vi "get queues.vi"(11 "error in (no error)":errorcluster) -> (4 "display queues":T1, 8 "disk queues":T1, 15 "error out":errorcluster)   [LabVIEW 2017]
uses:
  typedefs/queue cluster.ctl
  typedefs/reading queue.ctl
  typedefs/reading.ctl
  typedefs/readingType.ctl
  typedefs/magnetomter reading set.ctl
  popup panels/control panel globals.vi
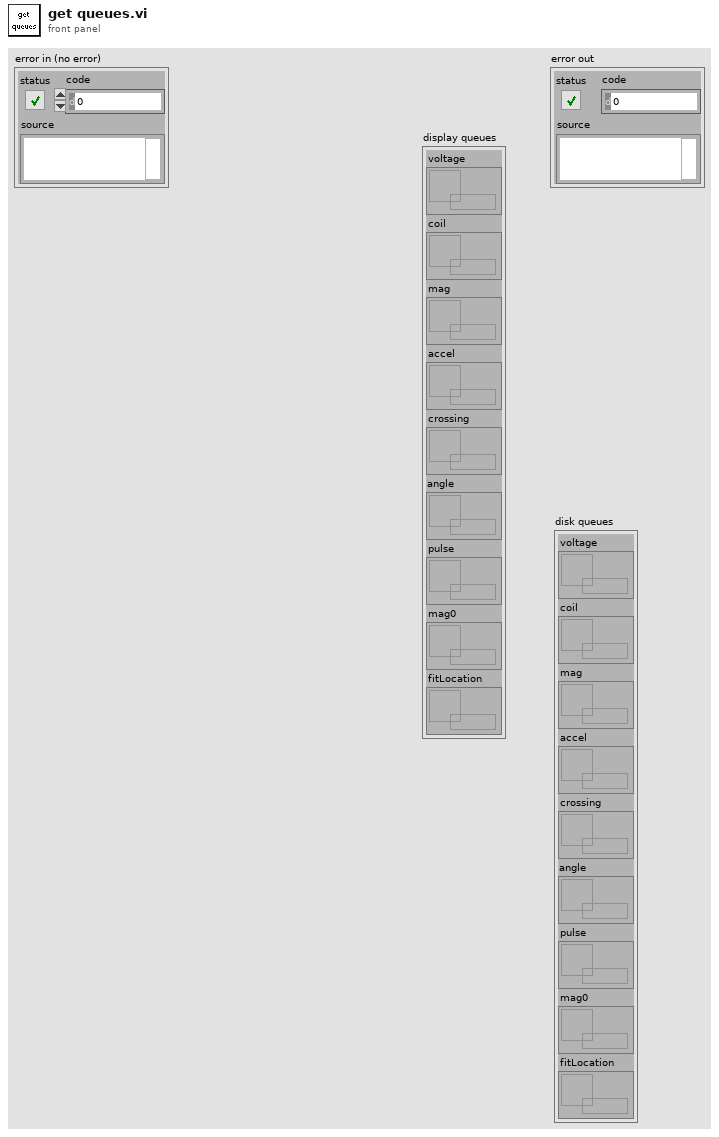
[diagram p1: front panel]
types:
  T1 = typedef "queue cluster.ctl" = cluster{"voltage":T2, "coil":T2, "mag":refnum<queue>, "accel":T2, "crossing":T2, "angle":T2, "pulse":T2, "mag0":T2, "fitLocation":T2}
  T2 = typedef "reading queue.ctl" = refnum<queue>
  T3 = typedef "magnetomter reading set.ctl" = cluster{"time":fxp<+,48,48>, "mag readings":cluster{"magnetometer index":dbl, "Bx":dbl, "By":dbl, "Bz":dbl, "magnetometer x":dbl, "magnetometer y":dbl}[]}
  T4 = typedef "reading.ctl" = cluster{"reading type":T5, "time":fxp<+,48,48>, "x":sgl, "y":sgl, "z":sgl, "XSUM":u8}
  T5 = typedef "readingType.ctl" = enum8{"SYNC", "DETVAL", "COILI", "MAGVEC", "ACCVEC", "CROSSING", "MAGVEC0", "MAGVEC1", "MAGVEC2", "MAGVEC3", "MAGVEC4", "MAGVEC5", "MAGVEC6", "MAGVEC7"}
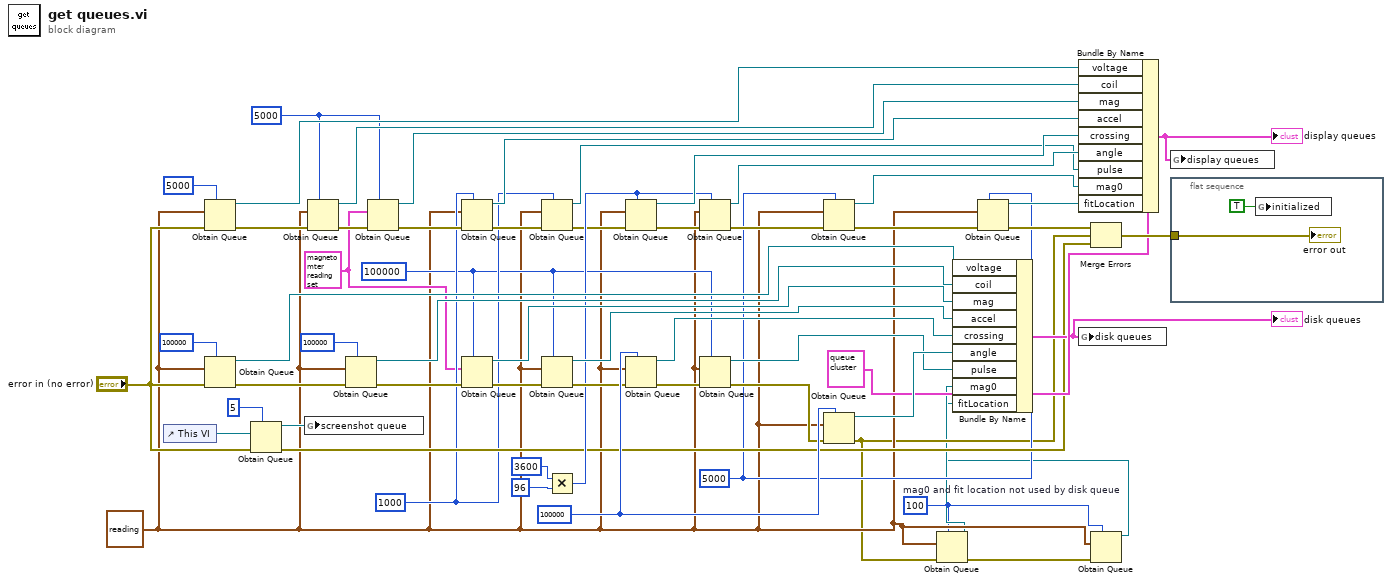
[diagram p0: block diagram]
diagram:
  w1 = 100  # mag0 and fit location not used by disk queue
  w7 = 5000 ("max queue size (-1, unlimited)")
  w13 = T3 {"time"=0.0, "mag readings"=[]} ("Magnetometer reading set")
  w32 = T1 {"voltage"=refnum, "coil"=refnum, "mag"=refnum, "accel"=refnum, "crossing"=refnum, "angle"=refnum, "pulse"=refnum, "mag0"=refnum, "fitLocation"=refnum} ("queue cluster")
  w36 = 100000 ("max queue size (-1, unlimited)")
  w15 = 100000 ("max queue size (-1, unlimited)")
  w19 = 1000 ("max queue size (-1, unlimited)")
  w6 = T4 {"reading type"=enum."SYNC", "time"=0.0, "x"=0.0, "y"=0.0, "z"=0.0, "XSUM"=0} ("reading3")
  w31 = 5000 ("max queue size (-1, unlimited)")
  n1 = control-ref of="This VI"() -> (w24:refnum<vi>)
  n2 = Obtain Queue(max queue size (-1, unlimited)=5000, element data type=w6, error in (no error)="error in (no error)") -> (queue out=w54:refnum<queue>, error out=w57:errorcluster)  [unwired: 2 in, 1 out]
  n3 = Obtain Queue(max queue size (-1, unlimited)=100000, element data type=w6, error in (no error)="error in (no error)") -> (queue out=w45:refnum<queue>, error out=w48:errorcluster)  [unwired: 2 in, 1 out]
  n4 = Obtain Queue(max queue size (-1, unlimited)=5, element data type=w24, error in (no error)="error in (no error)") -> (queue out=w22:refnum<queue>, error out=w23:errorcluster)  [unwired: 2 in, 1 out]
  n5 = global write "control panel globals.vi" "screenshot queue"(w22) -> ()
  n6 = Obtain Queue(max queue size (-1, unlimited)=w31, element data type=w6, error in (no error)=w57) -> (queue out=w53:refnum<queue>, error out=w56:errorcluster)  [unwired: 2 in, 1 out]
  n7 = Obtain Queue(max queue size (-1, unlimited)=100000, element data type=w6, error in (no error)=w48) -> (queue out=w44:refnum<queue>, error out=w47:errorcluster)  [unwired: 2 in, 1 out]
  n8 = Obtain Queue(max queue size (-1, unlimited)=w31, element data type=w13, error in (no error)=w56) -> (queue out=w52:refnum<queue>, error out=w55:errorcluster)  [unwired: 2 in, 1 out]
  n9 = Obtain Queue(max queue size (-1, unlimited)=w19, element data type=w6, error in (no error)=w55) -> (queue out=w51:refnum<queue>, error out=w21:errorcluster)  [unwired: 2 in, 1 out]
  n10 = Obtain Queue(max queue size (-1, unlimited)=w15, element data type=w13, error in (no error)=w47) -> (queue out=w43:refnum<queue>, error out=w46:errorcluster)  [unwired: 2 in, 1 out]
  n11 = Obtain Queue(max queue size (-1, unlimited)=w19, element data type=w6, error in (no error)=w21) -> (queue out=w18:refnum<queue>, error out=w20:errorcluster)  [unwired: 2 in, 1 out]
  n12 = Obtain Queue(max queue size (-1, unlimited)=w15, element data type=w6, error in (no error)=w46) -> (queue out=w42:refnum<queue>, error out=w33:errorcluster)  [unwired: 2 in, 1 out]
  n13 = Multiply(x=3600, y=96 ("max queue size (-1, unlimited)")) -> (x*y=w28:i32)
  n14 = Obtain Queue(max queue size (-1, unlimited)=w28, element data type=w6, error in (no error)=w20) -> (queue out=w40:refnum<queue>, error out=w39:errorcluster)  [unwired: 2 in, 1 out]
  n15 = Obtain Queue(max queue size (-1, unlimited)=w36, element data type=w6, error in (no error)=w33) -> (queue out=w35:refnum<queue>, error out=w17:errorcluster)  [unwired: 2 in, 1 out]
  n16 = Obtain Queue(max queue size (-1, unlimited)=w28, element data type=w6, error in (no error)=w39) -> (queue out=w37:refnum<queue>, error out=w12:errorcluster)  [unwired: 2 in, 1 out]
  n17 = Obtain Queue(max queue size (-1, unlimited)=w15, element data type=w6, error in (no error)=w17) -> (queue out=w14:refnum<queue>, error out=w16:errorcluster)  [unwired: 2 in, 1 out]
  n18 = Obtain Queue(max queue size (-1, unlimited)=w7, element data type=w6, error in (no error)=w12) -> (queue out=w10:refnum<queue>, error out=w11:errorcluster)  [unwired: 2 in, 1 out]
  n19 = Obtain Queue(max queue size (-1, unlimited)=w36, element data type=w6, error in (no error)=w16) -> (queue out=w34:refnum<queue>, error out=w5:errorcluster)  [unwired: 2 in, 1 out]
  n20 = Obtain Queue(max queue size (-1, unlimited)=w1, element data type=w6, error in (no error)=w5) -> (queue out=w3:refnum<queue>, error out=w4:errorcluster)  [unwired: 2 in, 1 out]
  n21 = Obtain Queue(max queue size (-1, unlimited)=w7, element data type=w6, error in (no error)=w11) -> (queue out=w8:refnum<queue>, error out=w9:errorcluster)  [unwired: 2 in, 1 out]
  n22 = Bundle By Name(cluster=w32, "voltage"=w54, "coil"=w53, "mag"=w52, "accel"=w51, "crossing"=w40, "angle"=w37, "pulse"=w18, "mag0"=w10, "fitLocation"=w8) -> (w29:T1)
  "display queues" <- w29
  n23 = Merge Errors(w9, w5, w23) -> (w41:errorcluster)
  n24 = Obtain Queue(max queue size (-1, unlimited)=w1, element data type=w6, error in (no error)=w4) -> (queue out=w2:refnum<queue>)  [unwired: 2 in, 2 out]
  n25 = Bundle By Name(cluster=w32, "voltage"=w45, "coil"=w44, "mag"=w43, "accel"=w42, "crossing"=w35, "angle"=w34, "pulse"=w14, "mag0"=w3, "fitLocation"=w2) -> (w30:T1)
  "disk queues" <- w30
  n26 = global write "control panel globals.vi" "disk queues"(w30) -> ()
  n27 = global write "control panel globals.vi" "display queues"(w29) -> ()
  n28 = flat-sequence {
    tunnel: w41 -> [w60]
    frame #0 {
      n29 = global write "control panel globals.vi" "initialized"(TRUE ("initialized")) -> ()
      "error out" <- w60
    }
  }
